vi "Agilent SNA Read Format.vi"(6 "Channel":i8=1 min=1 max=99 step=1, 7 "Agilent SNA":T1, 8 "error in (no error)":errorcluster, 11 "VISA Resource Names":T2) -> (0 "error out":errorcluster, 2 "Display Format":T3, 3 "dup VISA Resource Names":T2)   [LabVIEW 2011]
doc: "This VI for the HP 8753B is used to read the meausurement format.\n\n0 log magnitude\n1 phase\n2 delay\n3 Smith chart\n4 polar\n5 linear magnitude\n6 standing wave ratio\n7 real\n8 imaginary"
uses:
  tests/S Parameter/TypeDefs/SP Measurement Format.ctl
  TypeDefs/Agilent SNA VISA.ctl
  TypeDefs/Agilent SNA Instrument Info.ctl
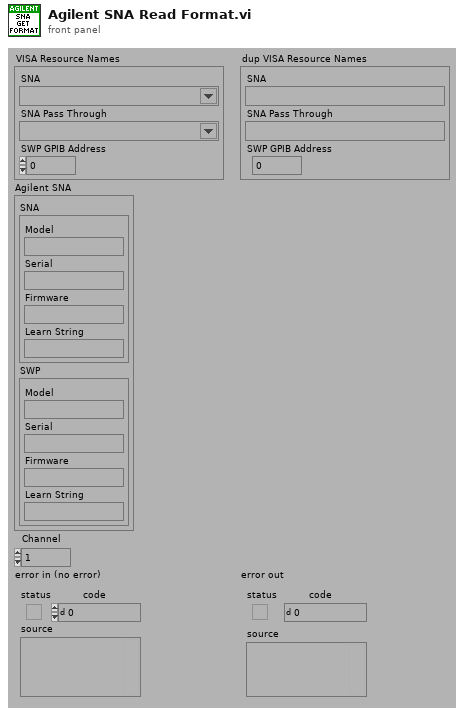
[diagram p1: front panel]
types:
  T1 = typedef "Agilent SNA Instrument Info.ctl" = cluster{"SNA":cluster{"Model":string, "Serial":string, "Firmware":string, "Learn String":string}, "SWP":cluster{"Model":string, "Serial":string, "Firmware":string, "Learn String":string}}
  T2 = typedef "Agilent SNA VISA.ctl" = cluster{"SNA":refnum<visa-resource-name>, "SNA Pass Through":refnum<visa-resource-name>, "SWP GPIB Address":i32}
  T3 = typedef "SP Measurement Format.ctl" = enum32{"Log Mag", "Phase", "Delay", "Smith (R+jX)", "Polar (Re/Im)", "Linear Mag", "SWR", "Real", "Imaginary", "Smith (Lin/Phase)", "Smith (Log/Phase)", "Smith (Real/Imag)", "Smith (G+jB)", "Polar (Lin/Phase)", "Polar (Log/Phase)", "Expanded Phase", "Positive Phase", "Inverted Smith", "Unwrapped Phase", "Power Out", "Power In", "Linear Mag/Phase", "Log Mag/Phase", "Real/Imaginary"}
  T4 = typedef "Agilent SNA Model.ctl" = enum16{"Not Supported", "8757X"}
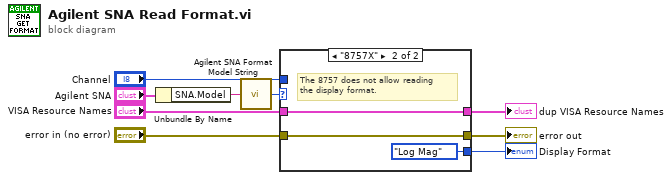
[diagram p0: block diagram]
diagram:
  n1 = Unbundle By Name("Agilent SNA") -> ("SNA.Model"=w1:string)
  n2 = call "Agilent SNA Format Model String.vi"("Model String"=w1) -> ("Model"=w4:T4)
  n3 = case shown="\"8757X\"" w4 {
    tunnel: "error in (no error)" -> [w10 w12]
    tunnel: [w10 w12] -> w8
    tunnel: [_ SP_Measurement_Format."Log Mag" ("Display Format")] -> w7
    tunnel: "VISA Resource Names" -> [w11 w13]
    tunnel: [w11 w13] -> w5
    tunnel: "Channel" -> [_ _]
    frame "Not Supported" {
    }
    frame "8757X" {
      # "The 8757 does not allow reading\nthe display format."
    }
  }
  "Display Format" <- w7
  "dup VISA Resource Names" <- w5
  "error out" <- w8
